vi "_TestMain.vi"() -> ()   [LabVIEW 2017]
uses:
  XTriPhaseGraph.xctl
panel:
  in  "stop":bool
  out "XTriPhaseGraph":waveform(dbl)[](xcontrol)
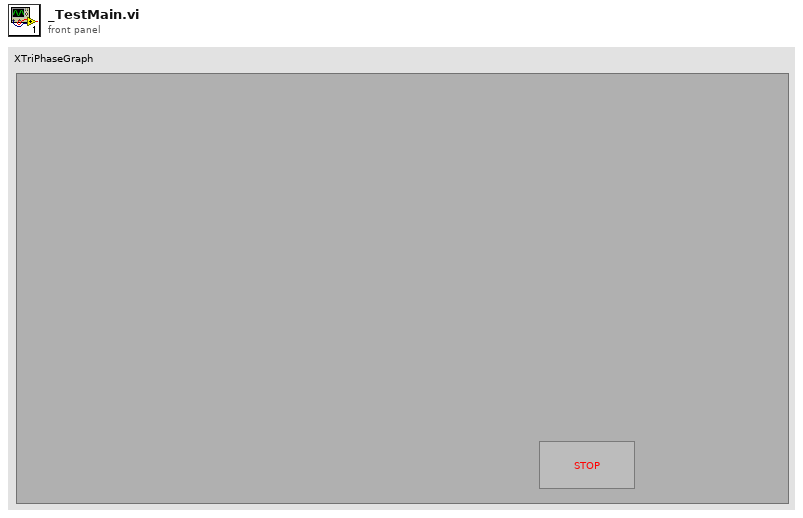
[diagram p1: front panel]
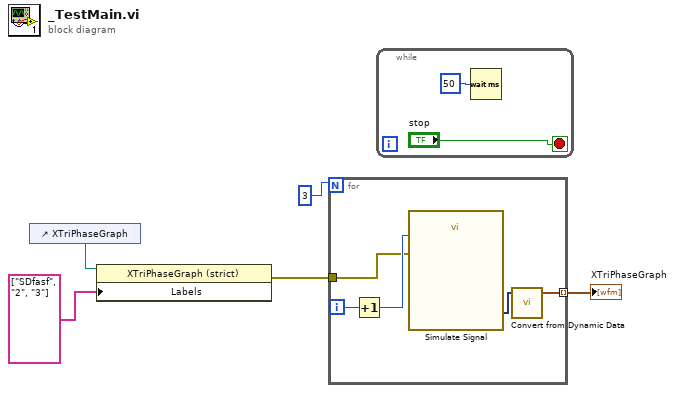
[diagram p0: block diagram]
diagram:
  n1 = control-ref of="XTriPhaseGraph"() -> (w1:refnum<vi>)
  n2 = property on="Property Node" class="XTriPhaseGraph (strict)"(reference=w1, "Labels"=string[] ["SDfasf", "2", "3"]) -> (error out=w3:errorcluster)  [unwired: 1 in, 1 out]
  n3 = for {
    N: 3 -> [_]
    tunnel: [w9] -> w5 mode=indexing
    tunnel: w3 -> [w6]
    i -> [w8]
    n4 = Increment(x=w8) -> (x+1=w7:i32)
    n5 = call "Simulate Signal"("Amplitude"=w7, "error in (no error)"=w6) -> ("Sine"=w10:dynamicdata)  [unwired: 12 in, 1 out]
    n6 = call "Convert from Dynamic Data"("Dynamic Data Type"=w10) -> ("Waveform"=w9:waveform(dbl))  [unwired: 3 in]
  }
  "XTriPhaseGraph" <- w5
  n7 = while {
    stop <- "stop" stop-if-true
    n8 = Wait (ms)(milliseconds to wait=u32 50) -> ()  [unwired: 1 out]
  }
